vi "Parse Snapshot.vi"(11 "String":string) -> (3 "Date time":string)   [LabVIEW 2015, in "NI_Azure_Blob.lvlib"]
uses:
  NI_Azure_Blob.lvlib
  <vilib>/Utility/error.llb/whitespace.ctl
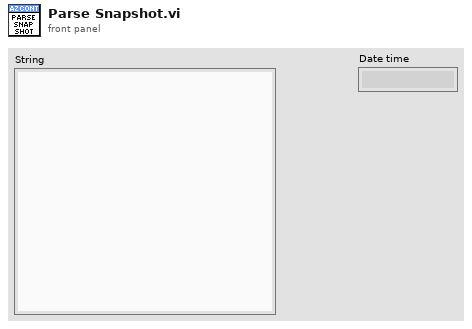
[diagram p1: front panel]
types:
  T1 = typedef "whitespace.ctl" = u16
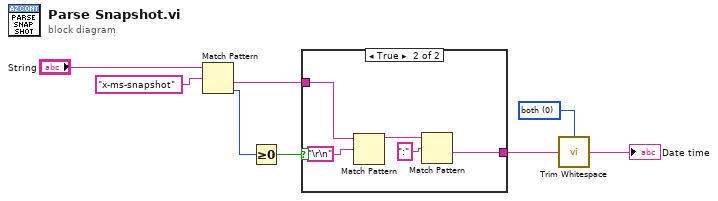
[diagram p0: block diagram]
diagram:
  w1 = T1 0 items=["both", "start of string", "end of string"] ("location (both)")
  n1 = Match Pattern(string="String", regular expression="x-ms-snapshot") -> (after substring=w5:string, offset past match=w6:i32)  [unwired: 1 in, 2 out]
  n2 = Greater Or Equal To 0?(x=w6) -> (x >= 0?=w4:bool)
  n3 = case shown="True" w4 {
    tunnel: w5 -> [_ w13]
    tunnel: [_ w9] -> w3
    frame False {
    }
    frame True {
      n4 = Match Pattern(string=w13, regular expression="\r\n") -> (before substring=w11:string)  [unwired: 1 in, 3 out]
      n5 = Match Pattern(string=w11, regular expression=":") -> (after substring=w9:string)  [unwired: 1 in, 3 out]
    }
  }
  n6 = call <vilib>:"Trim Whitespace.vi"("string"=w3, "location (both)"=w1) -> ("trimmed string"=→"Date time":string)
